vi "TSVPyFix.vi"(8 "error in (no error)":errorcluster, 11 "Path to text file":path) -> (0 "error out":errorcluster, 3 "Path to gleaned text file":path)   [LabVIEW 2016, in "VCL_2_DSC.lvclass"]
uses:
  VCL_2_DSC.lvclass
panel:
  out "standard error":string
  out "standard output":string
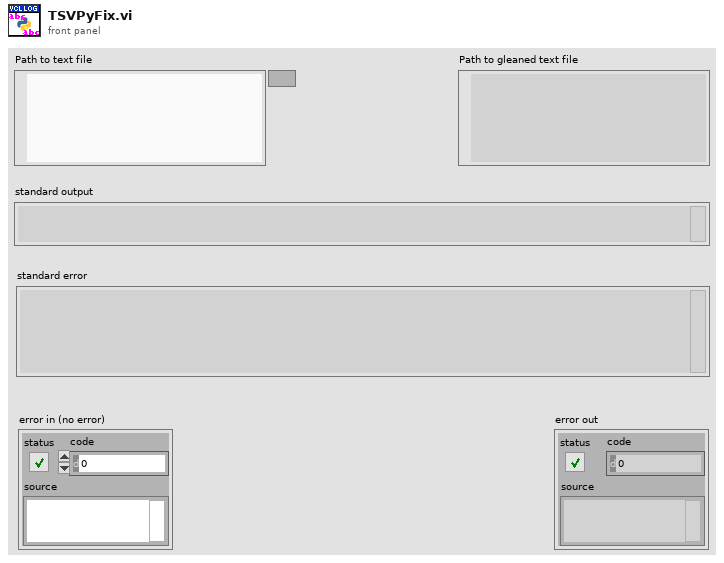
[diagram p1: front panel]
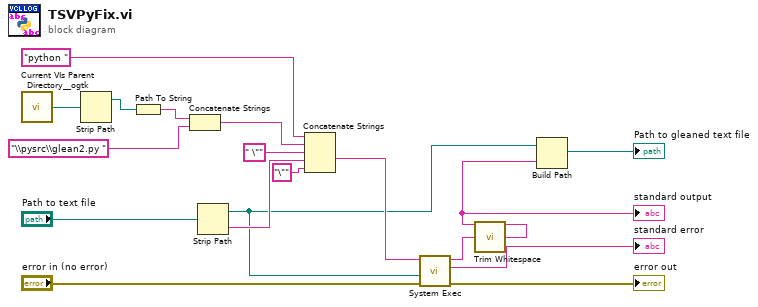
[diagram p0: block diagram]
diagram:
  n1 = call <userlib>:"Current VIs Parent Directory__ogtk.vi"() -> ("Parent Directory (+ Relative)"=w6:path)  [unwired: 5 in]
  n2 = Strip Path(path=w6) -> (stripped path=w5:path)  [unwired: 1 out]
  n3 = Path To String(path=w5) -> (string=w9:string)
  n4 = Concatenate Strings(w9, "\\pysrc\\glean2.py " ("full path to VCL_2_ASCII_CONVERTER.exe")) -> (w7:string)
  n5 = Strip Path(path="Path to text file") -> (stripped path=w4:path, name=w13:string)
  n6 = Concatenate Strings("python " ("command line"), w7, " \"" ("string"), w13, "\"" ("string")) -> (w12:string)
  n7 = call <vilib>:"System Exec.vi"("error in (no error)"="error in (no error)", "working directory"=w4, "command line"=w12) -> ("error out"=→"error out":errorcluster, "standard error"=→"standard error":string, "standard output"=w2:string)  [unwired: 5 in, 1 out]
  n8 = call <vilib>:"Trim Whitespace.vi"("string"=w2) -> ("trimmed string"=w1:string)  [unwired: 1 in]
  "standard output" <- w1
  n9 = Build Path(base path=w4, name or relative path=w1) -> (appended path=→"Path to gleaned text file":path)
